vi "receive header message.vi"(8 "error in (no error)":errorcluster, 11 "Channel in":refnum<class "Channel.lvclass">) -> (0 "error out":errorcluster, 3 "Channel out":refnum<class "Channel.lvclass">)   [LabVIEW 2018, in "Channel.lvclass"]
uses:
  Channel.lvclass
  Channel.lvclass/Channel.ctl
  Header content/Header content.lvclass
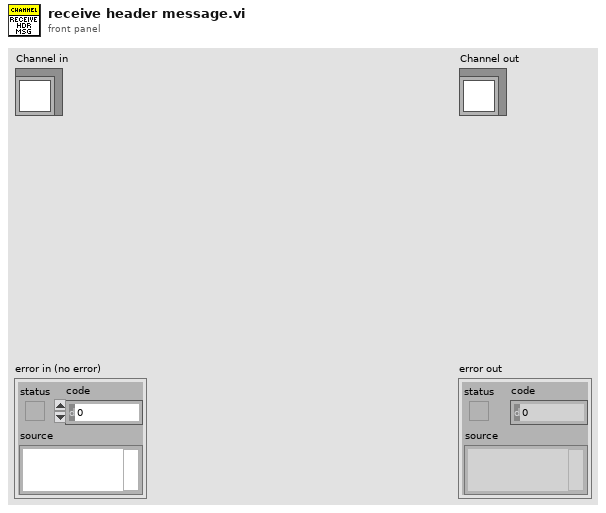
[diagram p1: front panel]
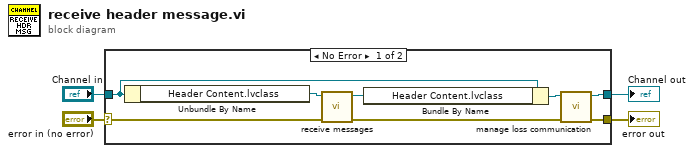
[diagram p0: block diagram]
diagram:
  n1 = case shown="No Error" "error in (no error)" {
    selector: "error in (no error)" -> [w11 w14]
    tunnel: [w5 w14] -> w3
    tunnel: [w6 w13] -> w1
    tunnel: "Channel in" -> [w10 w13]
    frame No Error {
      n2 = Unbundle By Name(w10) -> ("Header Content.lvclass"=w12:refnum<class "Header content.lvclass">)
      n3 = call "receive messages.vi"("error in (no error)"=w11, "Header content in"=w12) -> ("error out"=w7:errorcluster, "Header content out"=w9:refnum<class "Header content.lvclass">)  [unwired: 8 in]
      n4 = Bundle By Name(cluster=w10, "Header Content.lvclass"=w9) -> (w8:refnum<class "Channel.lvclass">)
      n5 = call "manage loss communication.vi"("error in (no error)"=w7, "Channel in"=w8) -> ("error out"=w5:errorcluster, "Channel out"=w6:refnum<class "Channel.lvclass">)  [unwired: 8 in]
    }
    frame Error {
    }
  }
  "error out" <- w3
  "Channel out" <- w1
